vi "Spectrum Scaling.vi"() -> ()   [LabVIEW 2015]
uses:
  Utility VIs/Math VIs/Linear to dB (scalar).vi
  Utility VIs/Math VIs/FFT x(t) to dB,Degrees (1D).vi
panel:
  out "Mag Spectrum":dbl[][](graph)
  out "Waveform Graph":dbl[](graph)
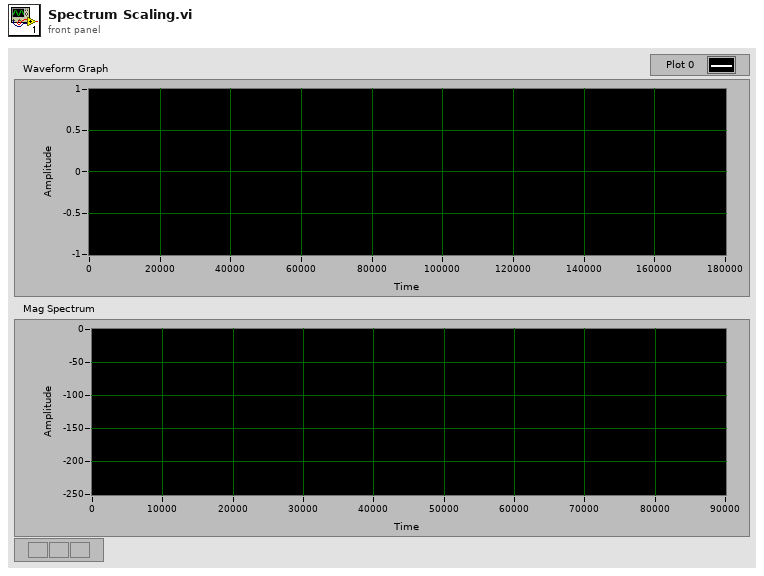
[diagram p1: front panel]
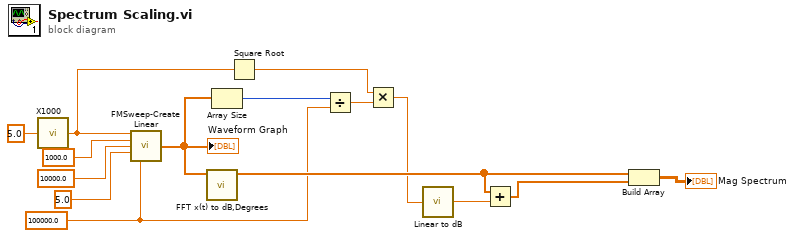
[diagram p0: block diagram]
diagram:
  w3 = 100000.0 ("Fs (Hz)")
  n1 = call "X1000.vi"("X"=5.0 ("Sweep Rate (Hz/s)")) -> ("X/1000"=w5:dbl)
  n2 = call "FMSweep-Create Linear.vi"("Sweep Rate (Hz/s)"=w5, "Fmin (Hz)"=1000.0, "Fmax (Hz)"=10000.0 ("Fmin (Hz)"), "Ramp (ms)"=5.0, "Fs (Hz)"=w3) -> ("Array"=w13:dbl[])  [unwired: 8 in, 2 out]
  "Waveform Graph" <- w13
  n3 = call-poly "FFT x(t) to dB,Degrees.vi"("X"=w13) -> ("+Freq. Mag of FFT (dB rms)"=w10:dbl[])  [unwired: 8 in, 2 out]
  n4 = Array Size(array=w13) -> (size(s)=w2:i32)
  n5 = Square Root(x=w5) -> (sqrt(x)=w8:dbl)
  n6 = Divide(x=w2, y=w3) -> (x/y=w1:dbl)
  n7 = Multiply(x=w8, y=w1) -> (x*y=w4:dbl)
  n8 = call-poly "Linear to dB.vi"("Linear"=w4) -> ("dB"=w12:dbl)
  n9 = Add(x=w10, y=w12) -> (x+y=w11:dbl[])
  n10 = Build Array(w10, w11) -> (→"Mag Spectrum":dbl[][])
